vi "_gStop.vi"(6 "op":T1=enum."set", 8 "error in (no error)":errorcluster, 10 "index(-1 for All)":i32=-1) -> (0 "error out":errorcluster, 2 "stop":bool)   [LabVIEW 2017, in "GSTOP.lvlib"]
uses:
  GSTOP.lvlib
  _def_oper.ctl
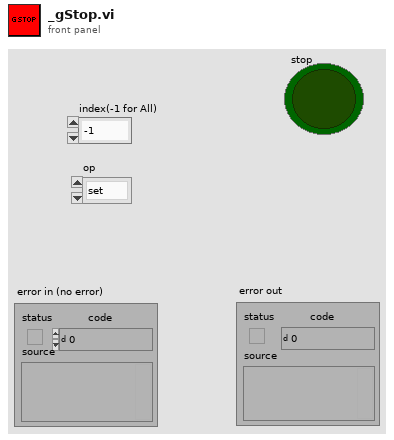
[diagram p1: front panel]
types:
  T1 = typedef "GSTOP.lvlib/_def_oper.ctl" = enum16{"init", "reset", "get", "set"}
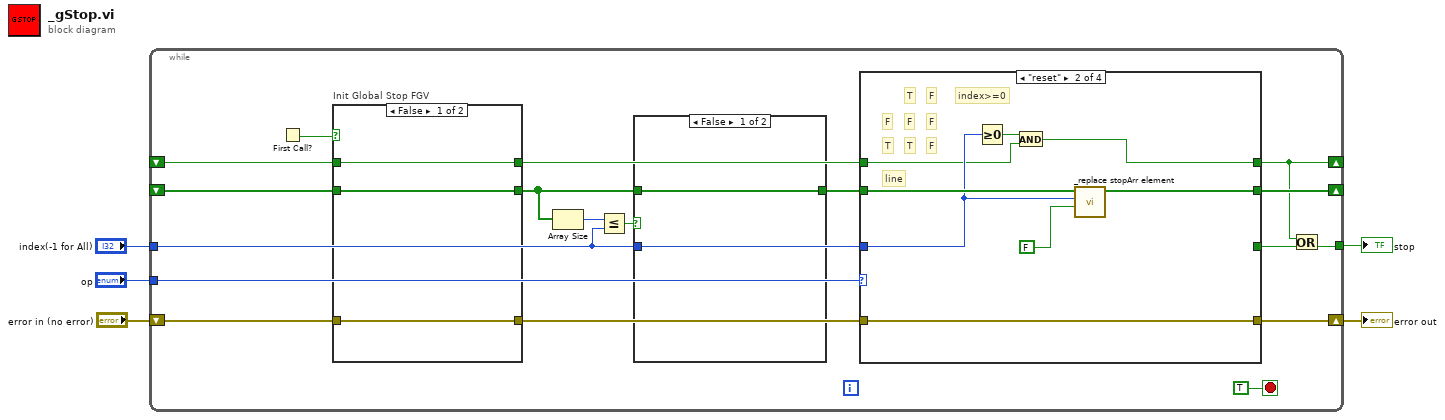
[diagram p0: block diagram]
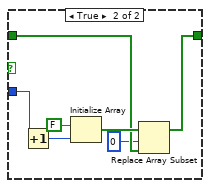
[diagram p2: hidden frame]
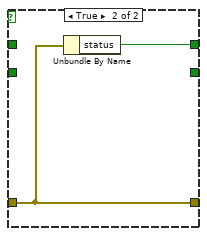
[diagram p3: hidden frame]
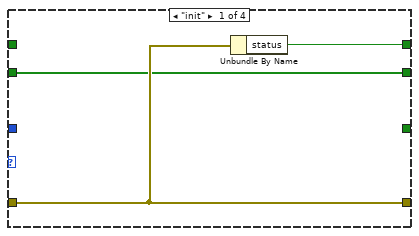
[diagram p4: hidden frame]
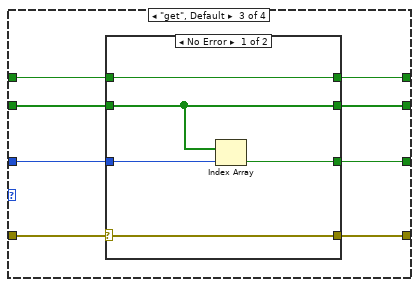
[diagram p5: hidden frame]
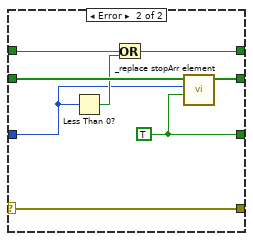
[diagram p6: hidden frame]
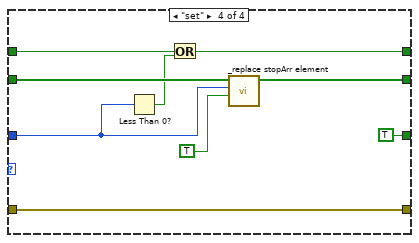
[diagram p7: hidden frame]
diagram:
  n1 = while {
    tunnel: "op" -> [w22]
    tunnel: "index(-1 for All)" -> [w6]
    shift-right: [w20] -> _
    shift-left: _ -> [w14]
    tunnel: [w13] -> w4
    shift-right: [w19] -> w2
    shift-left: "error in (no error)" -> [w17]
    shift-right: [w12] -> _
    shift-left: _ -> [w16]
    stop <- TRUE stop-if-true
    n2 = First Call?() -> (First Call?: T/F=w18:bool)
    n3 = case "Init Global Stop FGV" shown="False" w18 {
      tunnel: w17 -> [w32 w36]
      tunnel: w16 -> [w34 _]
      tunnel: [w34 w35] -> w15
      tunnel: w14 -> [w33 _]
      tunnel: [w33 _] -> w7
      tunnel: [w32 w36] -> w11
      frame False {
      }
      frame True {
        n4 = Unbundle By Name(w36) -> ("status"=w35:bool)
      }
    }
    n5 = Array Size(array=w7) -> (size(s)=w10:i32)
    n6 = Less Or Equal?(x=w10, y=w6) -> (x <= y?=w9:bool)
    n7 = case shown="False" w9 {
      tunnel: w6 -> [_ w30]
      tunnel: [w24 w26] -> w8
      tunnel: w7 -> [w24 w28]
      frame False {
      }
      frame True {
        n8 = Increment(x=w30) -> (x+1=w25:i32)
        n9 = Initialize Array(FALSE ("element"), w25) -> (w29:bool[])
        n10 = Replace Array Subset(array=w29, new element=w28, index=0) -> (w26:bool[])
      }
    }
    n11 = case shown="\"reset\"" w22 {
      tunnel: [_ _ w50 TRUE] -> w21
      tunnel: w6 -> [_ w43 w54 w72]
      tunnel: [w37 w46 w51 w74] -> w20
      tunnel: w8 -> [w37 w47 w55 w75]
      tunnel: [w38 w45 w53 w76] -> w19
      tunnel: w11 -> [w38 w45 w52 w76]
      tunnel: w15 -> [_ w41 w48 w70]
      tunnel: [w39 w40 w49 w69] -> w12
      frame "init" {
        n12 = Unbundle By Name(w38) -> ("status"=w39:bool)
      }
      frame "reset" {
        # "line"
        # "index>=0"
        # "F"
        # "F"
        # "T"
        # "T"
        # "F"
        # "F"
        # "F"
        # "T"
        n13 = Greater Or Equal To 0?(x=w43) -> (x >= 0?=w42:bool)
        n14 = And(x=w42, y=w41) -> (x .and. y?=w40:bool)
        n15 = call "_replace stopArr element.vi"("new element/subarray"=FALSE, "index"=w43, "Array in"=w47) -> ("Array out"=w46:bool[])  [unwired: 8 in]
      }
      frame "get", Default {
        n16 = case shown="No Error" w52 {
          selector: w52 -> [w58 w68]
          tunnel: [w60 w66] -> w50
          tunnel: w55 -> [w57 w67]
          tunnel: w54 -> [w59 w63]
          tunnel: [w58 w68] -> w53
          tunnel: [w57 w65] -> w51
          tunnel: [w56 w61] -> w49
          tunnel: w48 -> [w56 w62]
          frame No Error {
            n17 = Index Array(array=w57, index=w59) -> (element=w60:bool)
          }
          frame Error {
            w66 = TRUE
            n18 = Less Than 0?(x=w63) -> (x < 0?=w64:bool)
            n19 = Or(x=w62, y=w64) -> (x .or. y?=w61:bool)
            n20 = call "_replace stopArr element.vi"("new element/subarray"=w66, "index"=w63, "Array in"=w67) -> ("Array out"=w65:bool[])  [unwired: 8 in]
          }
        }
      }
      frame "set" {
        n21 = Less Than 0?(x=w72) -> (x < 0?=w71:bool)
        n22 = Or(x=w70, y=w71) -> (x .or. y?=w69:bool)
        n23 = call "_replace stopArr element.vi"("new element/subarray"=TRUE, "index"=w72, "Array in"=w75) -> ("Array out"=w74:bool[])  [unwired: 8 in]
      }
    }
    n24 = Or(x=w12, y=w21) -> (x .or. y?=w13:bool)
  }
  "stop" <- w4
  "error out" <- w2
